vi "FPGA Target Approach Retraction2(1).vi"() -> ()   [LabVIEW 2012]
uses:
  <vilib>/rvi/interface/RandomDataEmulation/nirviRandomDataFPGAFIFO.vi
  <vilib>/rvi/interface/RandomDataEmulation/niFpgaRandomDataHandleErrors.vi
  <vilib>/rvi/eio/common/nirviEmuTemplateMethod_errors.vi
  <vilib>/rvi/DataTransferAndStorage/Container/XNode/niFpgaContainer.xnode
  <vilib>/rvi/interface/RandomDataEmulation/nirviRandomDataFpgaReadWriteTemplate.vi
  <vilib>/eio/EIONode/EIONode.xnode
  <vilib>/rvi/Analysis/measure/butterworth/XNode/niFpgaButterworthFilter.xnode
panel:
  out "Ticks":i16
  in  "Data Acquisition Rate":i16
  out "HV/10":i16
  out "Tuning Fork Signal":fxp<+/-,24,17>
  out "FPGA Output Voltage":fxp<+/-,64,32>
  out "Z Fine Indicator":fxp<+/-,40,30>
  out "Counter Indicator":i32
  in  "Z Fine Output":fxp<+/-,40,30>
  in  "Counter Output":i32
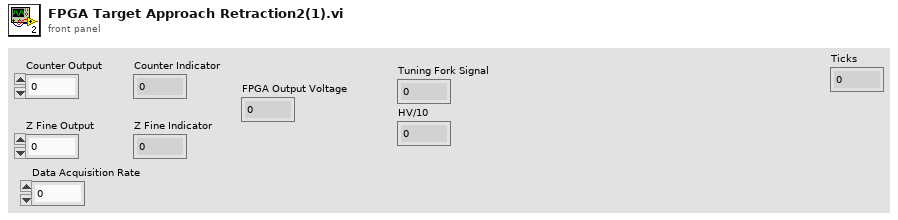
[diagram p1: front panel]
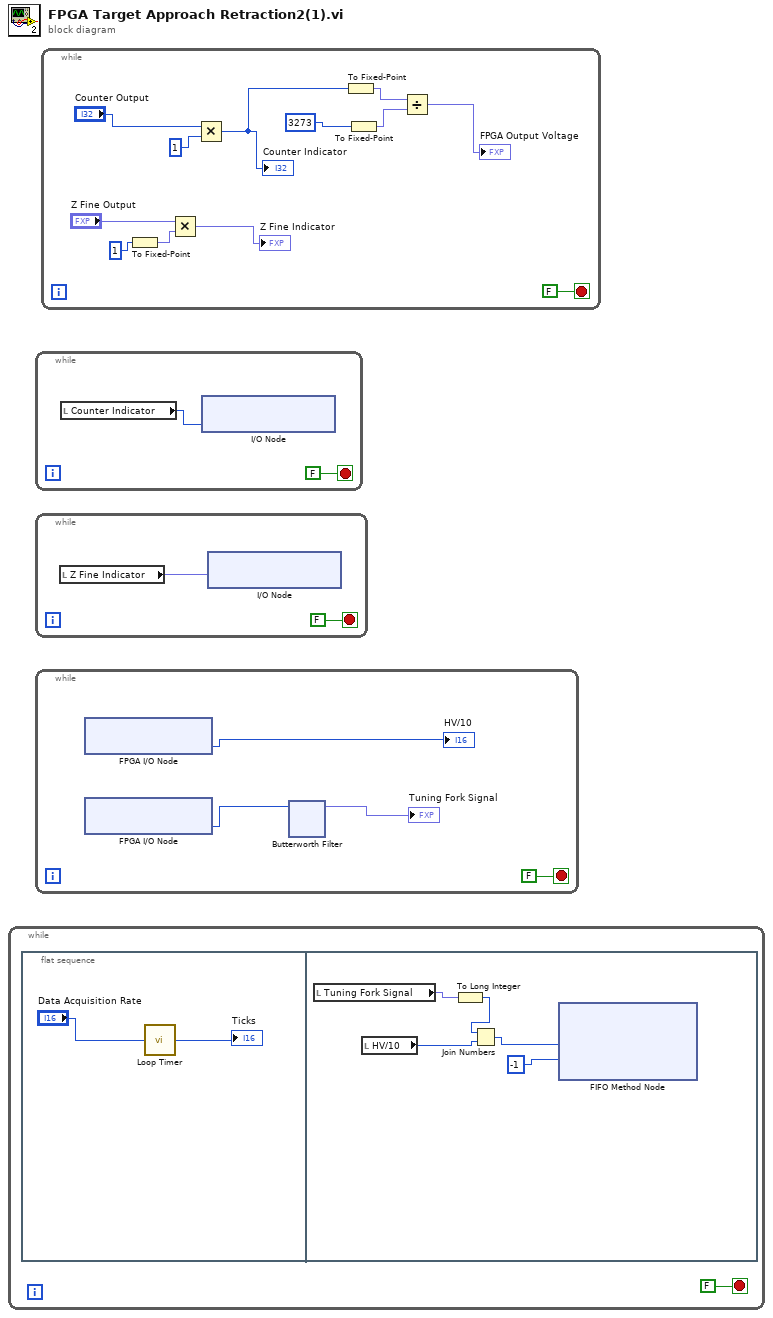
[diagram p0: block diagram]
diagram:
  n1 = while {
    stop <- FALSE stop-if-true
    n2 = flat-sequence {
      frame #0 {
        n3 = call "Loop Timer"("Count(uSec)"="Data Acquisition Rate") -> ("Tick Count(uSec)"=→"Ticks":u32)
      }
      frame #1 {
        n4 = local read "Tuning Fork Signal"() -> (w7:fxp<+/-,24,17>)
        n5 = local read "HV/10"() -> (w8:i16)
        n6 = To Long Integer(number=w7) -> (32bit integer=w6:i32)
        n7 = Join Numbers(hi=w6, lo=w8) -> ((hi.lo)=w5:u64)
        n8 = xnode ("FIFO Method Node")("Element"=w5, "Timeout"=i16 -1) -> ()  [unwired: 1 in, 2 out]
      }
    }
  }
  n9 = while {
    stop <- FALSE stop-if-true
    n10 = local read "Counter Indicator"() -> (w9:i32)
    n11 = xnode "I/O Node"("Connector0/AO7"=w9) -> ()  [unwired: 1 in, 1 out]
  }
  n12 = while {
    stop <- FALSE stop-if-true
    n13 = local read "Z Fine Indicator"() -> (w11:fxp<+/-,40,30>)
    n14 = xnode "I/O Node"("Connector0/AO2"=w11) -> ()  [unwired: 1 in, 1 out]
  }
  n15 = while {
    stop <- FALSE stop-if-true
    n16 = xnode "FPGA I/O Node"() -> ("Connector0/AI6"=→"HV/10":i16)  [unwired: 1 in, 1 out]
    n17 = xnode "FPGA I/O Node"() -> ("Connector0/AI7"=w15:i16)  [unwired: 1 in, 1 out]
    n18 = xnode "Butterworth Filter"("input data"=w15) -> ("output data"=→"Tuning Fork Signal":fxp<+/-,20,20>)  [unwired: 2 in]
  }
  n19 = while {
    stop <- FALSE stop-if-true
    n20 = To Fixed-Point(number=1) -> (fixed-point=w30:fxp<+/-,32,32>)  [unwired: 1 in]
    n21 = Multiply(x="Z Fine Output", y=w30) -> (x*y=→"Z Fine Indicator":fxp<+/-,64,62>)
    n22 = Multiply(x="Counter Output", y=1) -> (x*y=w28:i32)
    "Counter Indicator" <- w28
    n23 = To Fixed-Point(number=w28) -> (fixed-point=w27:fxp<+/-,32,32>)  [unwired: 1 in]
    n24 = To Fixed-Point(number=3273) -> (fixed-point=w26:fxp<+/-,32,32>)  [unwired: 1 in]
    n25 = Divide(x=w27, y=w26) -> (x/y=→"FPGA Output Voltage":fxp<+/-,64,33>)
  }
